vi "NiFPGA Write.vi"   [LabVIEW 2010, in "FPGA Interface Wrapper.lvlib"]
uses:
  <userlib>/_FPGA Interface Advanced Tools/FPGA Interface Wrapper/FPGA Interface Wrapper.lvlib
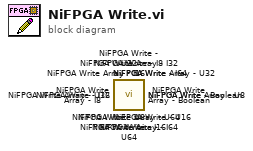
[diagram p0: block diagram]
diagram:
  n1 = call <userlib>:"NiFPGA Write Array - U64.vi"() -> ()  [unwired: 10 in, 2 out]
  n2 = call <userlib>:"NiFPGA Write Array - U32.vi"() -> ()  [unwired: 10 in, 2 out]
  n3 = call <userlib>:"NiFPGA Write Array - U16.vi"() -> ()  [unwired: 10 in, 2 out]
  n4 = call <userlib>:"NiFPGA Write Array - U8.vi"() -> ()  [unwired: 10 in, 2 out]
  n5 = call <userlib>:"NiFPGA Write Array - I64.vi"() -> ()  [unwired: 10 in, 2 out]
  n6 = call <userlib>:"NiFPGA Write Array - I32.vi"() -> ()  [unwired: 10 in, 2 out]
  n7 = call <userlib>:"NiFPGA Write Array - I16.vi"() -> ()  [unwired: 10 in, 2 out]
  n8 = call <userlib>:"NiFPGA Write Array - I8.vi"() -> ()  [unwired: 10 in, 2 out]
  n9 = call <userlib>:"NiFPGA Write Array - Boolean.vi"() -> ()  [unwired: 10 in, 2 out]
  n10 = call <userlib>:"NiFPGA Write - U64.vi"() -> ()  [unwired: 10 in, 2 out]
  n11 = call <userlib>:"NiFPGA Write - U32.vi"() -> ()  [unwired: 10 in, 2 out]
  n12 = call <userlib>:"NiFPGA Write - U16.vi"() -> ()  [unwired: 10 in, 2 out]
  n13 = call <userlib>:"NiFPGA Write - U8.vi"() -> ()  [unwired: 10 in, 2 out]
  n14 = call <userlib>:"NiFPGA Write - I64.vi"() -> ()  [unwired: 10 in, 2 out]
  n15 = call <userlib>:"NiFPGA Write - I32.vi"() -> ()  [unwired: 10 in, 2 out]
  n16 = call <userlib>:"NiFPGA Write - I16.vi"() -> ()  [unwired: 10 in, 2 out]
  n17 = call <userlib>:"NiFPGA Write - I8.vi"() -> ()  [unwired: 10 in, 2 out]
  n18 = call <userlib>:"NiFPGA Write - Boolean.vi"() -> ()  [unwired: 10 in, 2 out]
